vi "xPCErrorMsg.vi"(1 "error number":i32) -> (0 "ErrorMsg":string)   [LabVIEW 2018]
uses:
  XPCAPI.DLL
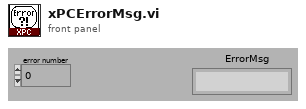
[diagram p1: front panel]
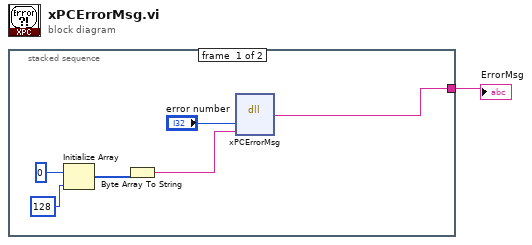
[diagram p0: block diagram]
diagram:
  n1 = stacked-sequence {
    tunnel: [w6 _] -> w1
    frame #0 {
      n2 = Initialize Array(u8 0 ("Element Data"), 128 ("Dimension Size")) -> (w3:u8[])
      n3 = Byte Array To String(unsigned byte array=w3) -> (string=w2:string)
      n4 = dll-call lib="PTH2mabs CUsers\nyuchengxinDesktop液压实验台11.16终结版液压实验台11.16终结版\nxpcapi.dll" fn="xPCErrorMsg"("port"="error number", "name"=w2) -> (w6:string)  [unwired: 5 in, 2 out]
    }
    frame #1 {
    }
  }
  "ErrorMsg" <- w1
